vi "PKG_IMC_CmpPolarVal.vi"(9 "inPort":i32, 10 "newpolar":i32, 11 "oldpolar":u32) -> (3 "function return":u32)   [LabVIEW 2011, in "IMC_Pkg4xxx.lvlib"]
doc: "PKG_IMC_CmpPolarVal(unsigned int oldpolar, int newpolar, int inPort);"
uses:
  IMC_Pkg4xxx.lvlib
  IMC_Pkg4xxx.dll
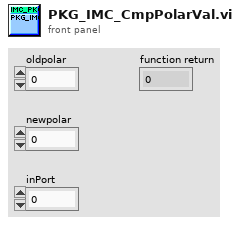
[diagram p1: front panel]
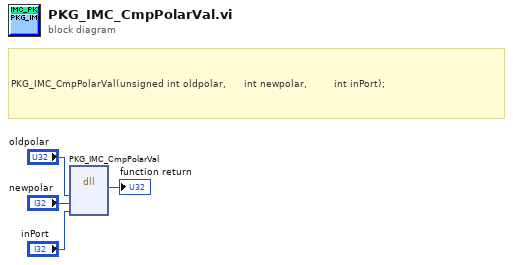
[diagram p0: block diagram]
diagram:
  # "PKG_IMC_CmpPolarVal(unsigned int oldpolar, \t\t\t\t\tint newpolar,\t\t\t\t\t\t\t\t\tint inPort);"
  n1 = dll-call lib="PTH1mabs F光盘刻录\niMC MotionIMCNet_V4.0IMCAppincLabviewIMC_PKG4xxxIMC_PKG4xxx\nIMC_Pkg4xxx.*" fn="PKG_IMC_CmpPolarVal"("oldpolar"="oldpolar", "newpolar"="newpolar", "inPort"="inPort") -> (→"function return":u32)  [unwired: 6 in, 2 out]
